vi "DinnerMenu_Create.vi"(8 "Error In":errorcluster, 11 "reference in":refnum<class "DinnerMenu.lvclass">) -> (0 "Error Out":errorcluster, 3 "reference out":refnum<class "DinnerMenu.lvclass">)   [LabVIEW 2020, in "DinnerMenu.lvclass"]
uses:
  DinnerMenu.lvclass
  Menu_class/Menu.lvclass
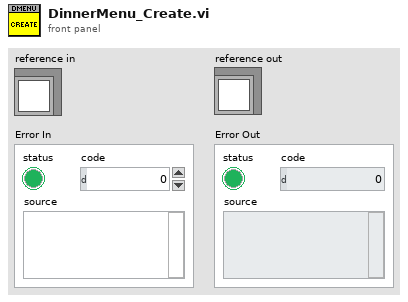
[diagram p1: front panel]
types:
  T1 = typedef "DinnerMenu.lvclass/ObjectAttributes.ctl" = cluster{"Max":i32, "_count":i32, "_items":refnum<class "Menu.lvclass">[], "Items":refnum<class "IEnumerable.lvclass">}
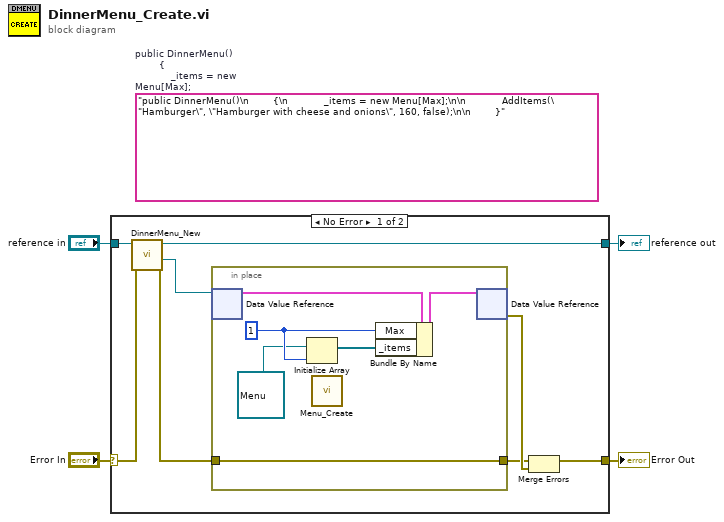
[diagram p0: block diagram]
diagram:
  (unwired) "public DinnerMenu()\n        {\n            _items = new Menu[Max];\n\n            AddItems(\"Hamburger\", \"Hamburger with cheese and onions\", 160, false);\n\n        }"  # public DinnerMenu()         {             _items = new Menu[Max];              AddItems("Hamburger", "Hamburger with cheese and onions", 160, false);          }
  n1 = case shown="No Error" "Error In" {
    selector: "Error In" -> [w11 w20]
    tunnel: [w5 w20] -> w3
    tunnel: "reference in" -> [w12 w19]
    tunnel: [w10 w19] -> w1
    frame No Error {
      n2 = call "DinnerMenu_New.vi"("error in (no error)"=w11, "reference in"=w12) -> ("error out"=w7:errorcluster, "DVRRefOut"=w8:refnum<data-value>, "reference out"=w10:refnum<class "DinnerMenu.lvclass">)  [unwired: 6 in, 1 out]
      n3 = in-place {
        in-place-border: w7 -> [w16]
        in-place-border: [w16] -> w6
        w15 = 1 ("Max")
        n4 = in-place-dvr #1(w8) -> (w17:T1)  [unwired: 1 out]
        n5 = Initialize Array(refnum<class "Menu.lvclass"> refnum ("Menu"), w15) -> (w14:refnum<class "Menu.lvclass">[])
        n6 = call "Menu_Create.vi"() -> ()  [unwired: 10 in, 2 out]
        n7 = Bundle By Name(cluster=w17, "Max"=w15, "_items"=w14) -> (w18:T1)
        n8 = in-place-dvr #1(w18) -> (w9:errorcluster)  [unwired: 1 out]
      }
      n9 = Merge Errors(w6, w9) -> (w5:errorcluster)
    }
    frame Error {
      # "VI-TechBaseTemplate_Simple_4x4x4"
    }
  }
  "Error Out" <- w3
  "reference out" <- w1
